vi "RefToValue.vi"   [LabVIEW 2013]
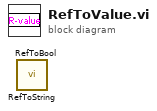
[diagram p0: block diagram]
diagram:
  n1 = call "RefToString.vi"() -> ()  [unwired: 6 in, 2 out]
  n2 = call "RefToBool.vi"() -> ()  [unwired: 6 in, 2 out]
